vi "Build Roll Maneuver.vi"(10 "Roll":T1, 11 "Timestep(ms)":i32=100) -> (0 "Total Time":i32, 1 "Angle Array":dbl[](array[numeric]), 2 "Y Array":dbl[](array[numeric]), 3 "X Array":dbl[](array[numeric]))   [LabVIEW 2013]
uses:
  Common Code/Dashboard UDP/Roll Maneuver.ctl
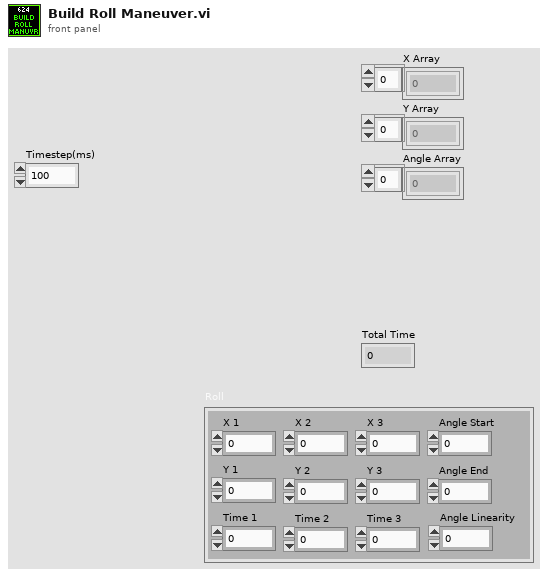
[diagram p1: front panel]
types:
  T1 = typedef "Roll Maneuver.ctl" = cluster{"X 1":dbl, "Y 1":dbl, "Y 2":dbl, "X 2":dbl, "Y 3":dbl, "X 3":dbl, "Time 1":i32, "Time 2":i32, "Time 3":i32, "Angle Start":dbl, "Angle End":dbl, "Angle Linearity":dbl}
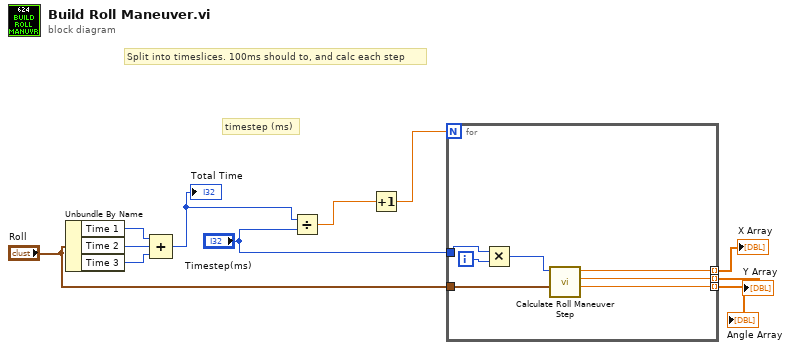
[diagram p0: block diagram]
diagram:
  # "timestep (ms)"
  # "Split into timeslices. 100ms should to, and calc each step"
  n1 = Unbundle By Name("Roll") -> ("Time 1"=w11:i32, "Time 2"=w10:i32, "Time 3"=w9:i32)
  n2 = Compound Arithmetic op=ADD(w11, w10, w9) -> (w4:i32)
  "Total Time" <- w4
  n3 = Divide(x=w4, y="Timestep(ms)") -> (x/y=w1:dbl)
  n4 = Increment(x=w1) -> (x+1=w2:dbl)
  n5 = for {
    N: w2 -> [_]
    tunnel: "Roll" -> [w17]
    tunnel: [w15] -> w7 mode=indexing
    tunnel: [w14] -> w6 mode=indexing
    tunnel: [w13] -> w5 mode=indexing
    tunnel: "Timestep(ms)" -> [w12]
    i -> [w18]
    n6 = Multiply(x=w12, y=w18) -> (x*y=w16:i32)
    n7 = call "Calculate Roll Maneuver Step.vi"("Roll"=w17, "Time"=w16) -> ("Angle"=w13:dbl, "Y"=w14:dbl, "X"=w15:dbl)  [unwired: 6 in, 1 out]
  }
  "X Array" <- w7
  "Y Array" <- w6
  "Angle Array" <- w5
